vi "Main.vi"(10 "Productos Subpanel":refnum<vi>, 11 "Module Admin":refnum<class "Delacor_lib_QMH_Module Admin.lvclass">) -> ()   [LabVIEW 2020, in "Producto.lvlib"]
doc: "This template is based off of the Queued Message Handler design pattern and the Queued Message Handler project template that ships with LabVIEW.\n\nThe main difference is that the queue is private to this module and communication between modules is performed via Broadcast and Request events.\n\nRequest events are wrapped in public API methods and are handled in the Event Handling Loop (EHL) of this VI. Any module can register for Broadcast events sent by this module. The EHL generates messages based on user interface actions.\n\nThe Message Handling Loop (MHL) processes messages generated by the EHL, or by other messages. The messages are string values, so new messages can be added easily to the Message Cases case structure in the MHL. Each message cluster can also provide an optional value for Message Data, which is a variant that can be converted to whatever message-specific data is required.\n_____\nBased on Delacor QMH Project Template 5.0.0.82."
uses:
  Producto.lvlib
  <vilib>/Delacor/Delacor QMH/Libraries/Module Admin_class/Delacor_lib_QMH_Module Admin.lvclass
  Module Data--cluster.ctl
  Stop Argument--cluster.ctl
  <vilib>/Delacor/Delacor QMH/Libraries/Message Queue_class/Delacor_lib_QMH_Message Queue.lvclass/Delacor_lib_QMH_Message Queue.ctl
  <vilib>/Delacor/Delacor QMH/Libraries/Module Admin_class/Delacor_lib_QMH_Module Admin.lvclass/Delacor_lib_QMH_Module Admin.ctl
  Set Products Argument--cluster.ctl
  Actualizar inventario Argument--cluster.ctl
  <vilib>/Utility/miscctls.llb/LVPointTypeDef.ctl
  <vilib>/Delacor/Delacor QMH/Libraries/Message Queue_class/Delacor_lib_QMH_Enqueue Message (Single).vi
  <vilib>/Delacor/Delacor QMH/Libraries/Module Admin_class/Delacor_lib_QMH_Get External Launch.vi
  <vilib>/Utility/error.llb/Error Cluster From Error Code.vi
  <vilib>/ErrorRing/Error Ring.xnode
  <vilib>/Delacor/Delacor QMH/Libraries/Message Queue_class/Delacor_lib_QMH_Message Queue.lvclass
  SQLLITEDATABASE/DataBaseSQLlite.lvlib
  Monedas/Monedas.lvlib
panel:
  in  "COMPRAR BUTONN":bool
  in  "Multicolumn Listbox":i32(listbox)
  out "error out":errorcluster
  out "Status":string
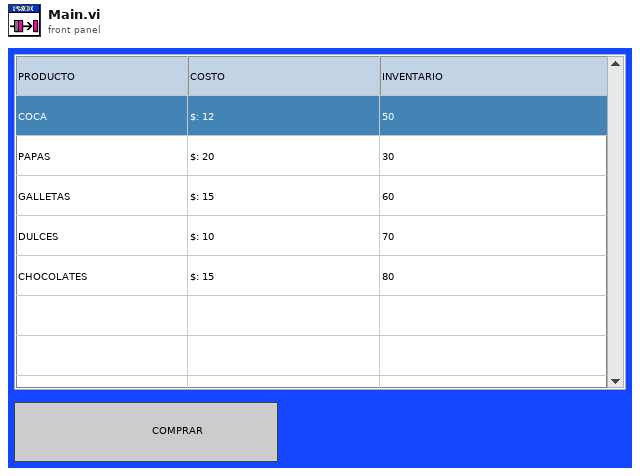
[diagram p1: front panel]
types:
  T1 = typedef "Monedas.lvlib/Broadcast Events--cluster.ctl" = cluster{"Module Did Init":refnum<user-event>, "Status Updated":refnum<user-event>, "Error Reported":refnum<user-event>, "Module Did Stop":refnum<user-event>, "Update Module Execution Status":refnum<user-event>}
  T2 = typedef "Producto.lvlib/Request Events--cluster.ctl" = cluster{"Stop Module":refnum<user-event>, "Show Panel":refnum<user-event>, "Hide Panel":refnum<user-event>, "Get Module Execution Status":refnum<user-event>, "Show Diagram":refnum<user-event>, "Set Products":refnum<user-event>, "Actualizar inventario":refnum<user-event>}
  T3 = typedef "Producto.lvlib/Module Data--cluster.ctl" = cluster{"Status":string, "PRODUCTOS EN Array":cluster{"PRODUCTO":string, "COSTO":dbl, "INVENTARIO":dbl}[], "MCListbox Refnum":refnum<vi>, "items":string[][]}
  T4 = enum32{"invalid lock state", "Not Locked", "Locked (No Password)", "Password-protected"}
  T5 = typedef "Producto.lvlib/Stop Argument--cluster.ctl" = cluster{"Origin":string, "Exit via Stop Module Req?":bool, "Wait for Module to stop?":bool}
  T6 = typedef "Producto.lvlib/Set Products Argument--cluster.ctl" = cluster{"Array":string[][]}
  T7 = typedef "Producto.lvlib/Actualizar inventario Argument--cluster.ctl" = cluster{"Boolean":bool, "Multicolumn Listbox":i32}
  T8 = typedef "LVPointTypeDef.ctl" = cluster{"Horizontal":i16, "Vertical":i16}
  T9 = enum32{"Invalid", "Standard", "Closed", "Hidden", "Minimized", "Maximized"}
  T10 = typedef "ProductInvenmtarytyppedef.ctl" = cluster{"PRODUCTO":string, "COSTO":dbl, "INVENTARIO":dbl}
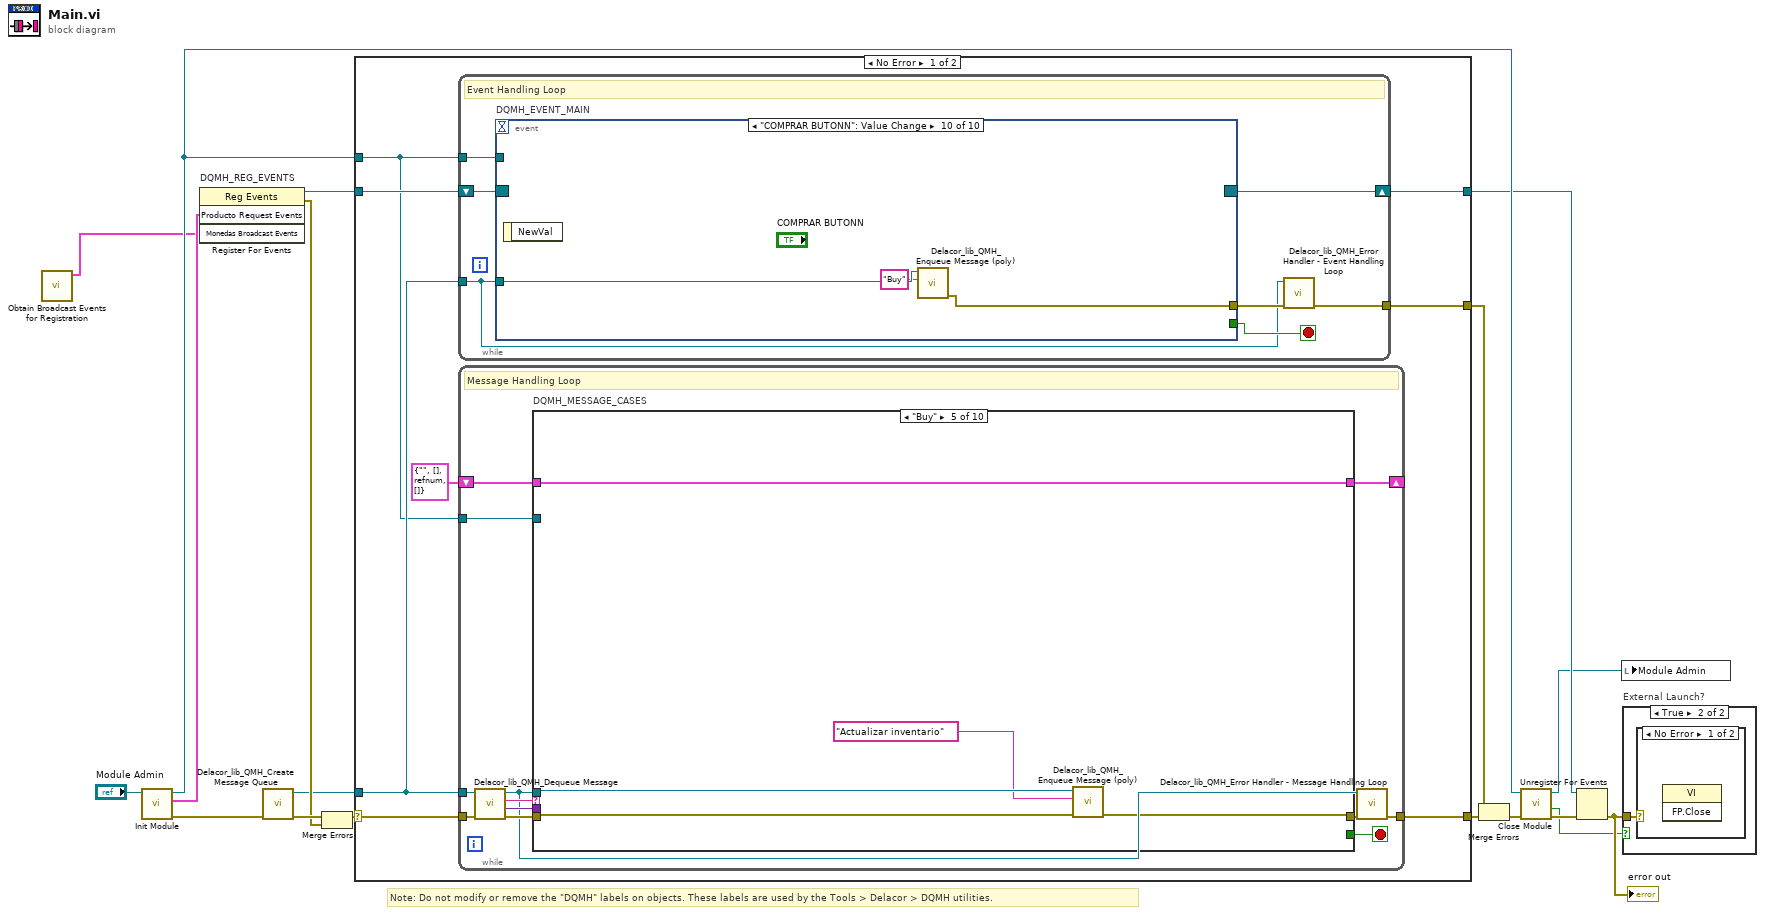
[diagram p0: block diagram]
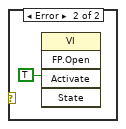
[diagram p3: hidden frame]
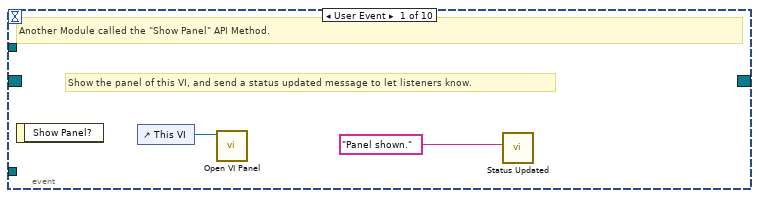
[diagram p4: hidden frame]
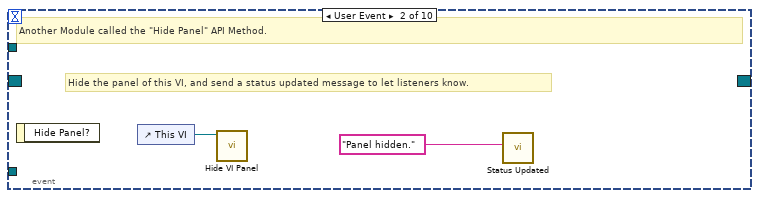
[diagram p5: hidden frame]
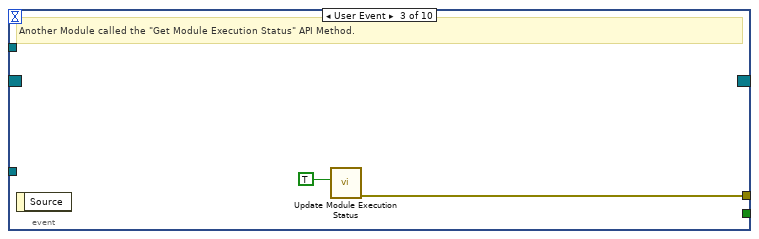
[diagram p6: hidden frame]
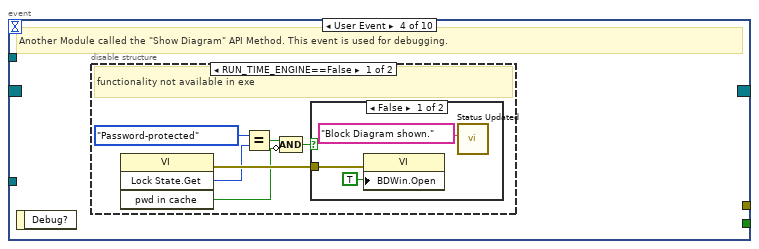
[diagram p7: hidden frame]
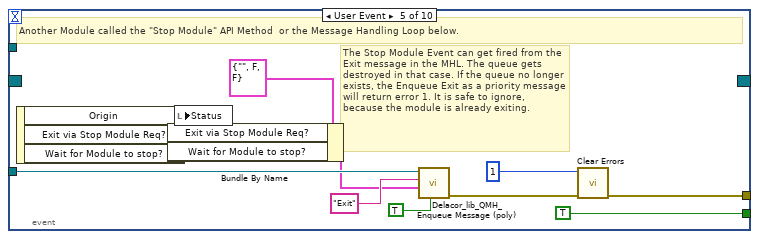
[diagram p10: hidden frame]
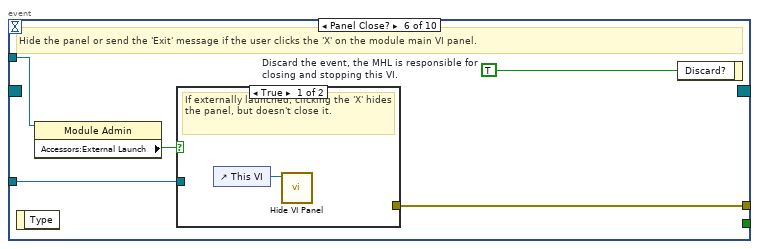
[diagram p11: hidden frame]
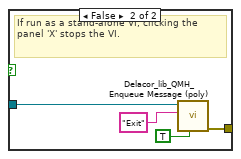
[diagram p12: hidden frame]
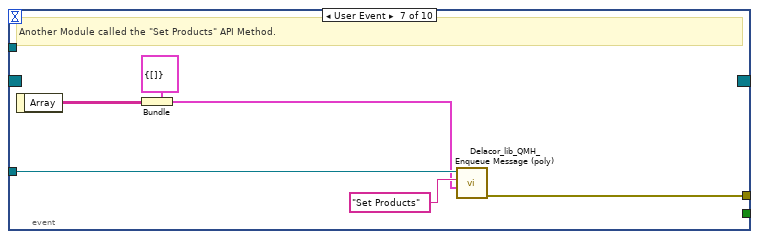
[diagram p13: hidden frame]
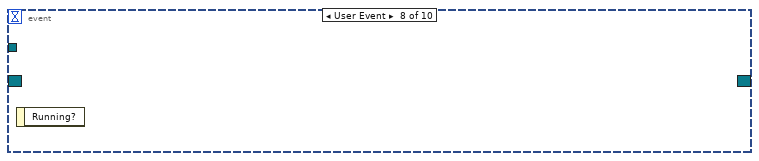
[diagram p14: hidden frame]
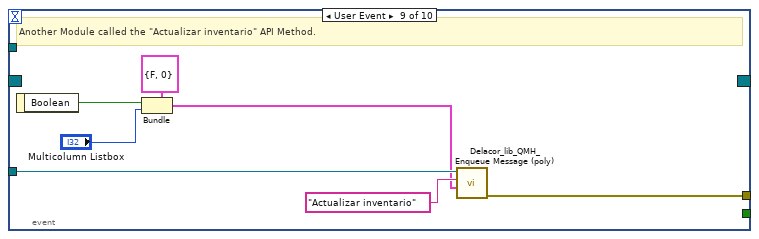
[diagram p15: hidden frame]
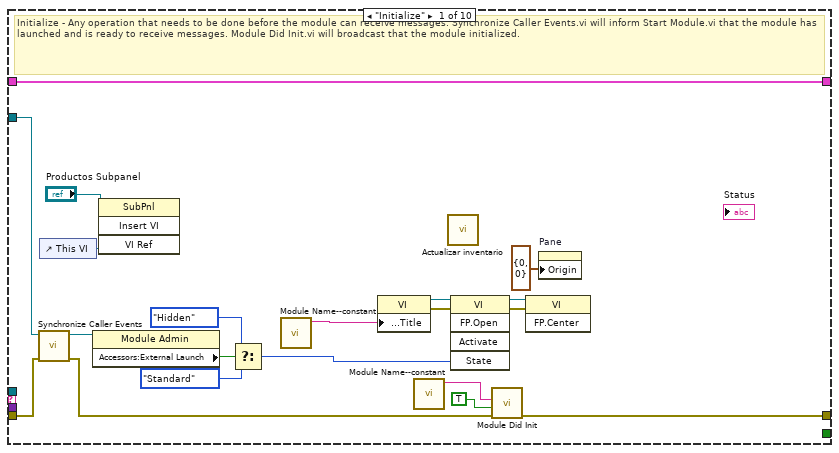
[diagram p16: hidden frame]
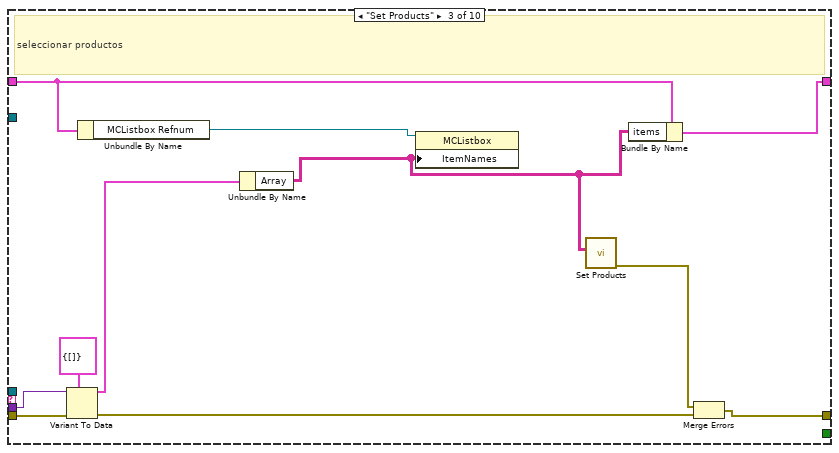
[diagram p18: hidden frame]
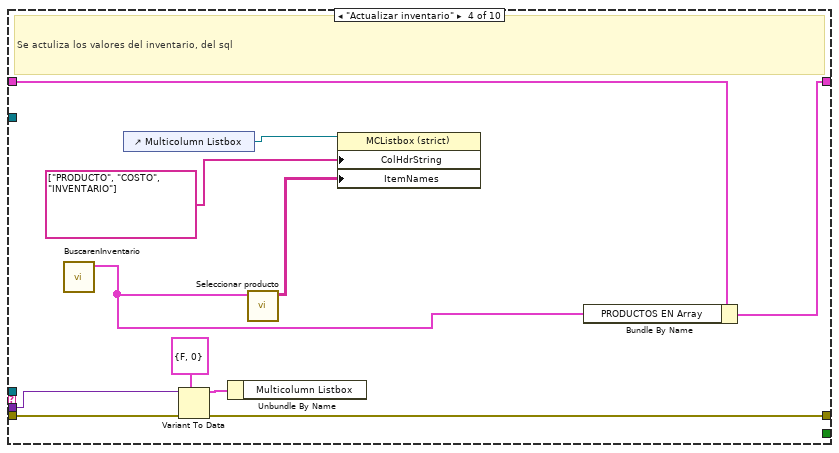
[diagram p19: hidden frame]
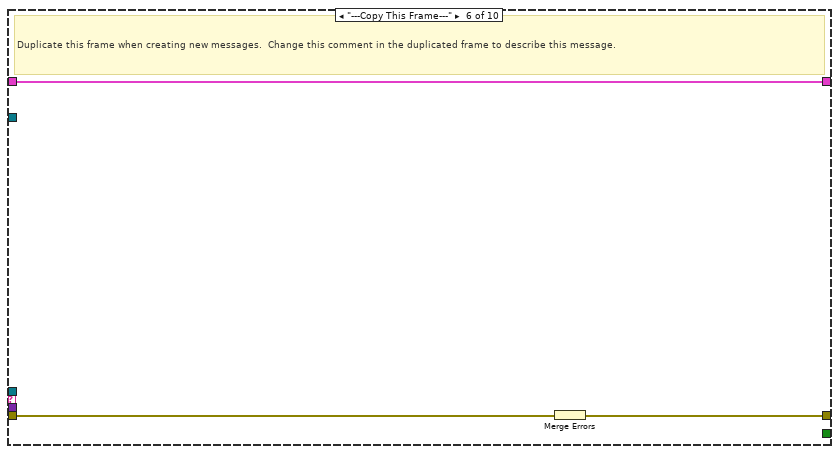
[diagram p20: hidden frame]
diagram:
  # "Note: Do not modify or remove the \"DQMH\" labels on objects. These labels are used by the Tools > Delacor > DQMH utilities."
  n1 = call "Obtain Broadcast Events for Registration.vi"() -> ("Monedas Broadcast Events"=w1:T1)  [unwired: 9 in, 2 out]
  n2 = call "Init Module.vi"("Singleton Module Admin in"="Module Admin") -> ("error out"=w17:errorcluster, "Producto Request Events"=w6:T2, "Singleton Module Admin out"=w9:refnum<class "Delacor_lib_QMH_Module Admin.lvclass">)  [unwired: 8 in]
  n3 = register-events "DQMH_REG_EVENTS"(w6, w1) -> (reference out=w7:refnum<event-registration>, error out=w10:errorcluster)  [unwired: 2 in]
  n4 = call <vilib>:"Delacor_lib_QMH_Create Message Queue.vi"("error in (no error)"=w17) -> ("error out"=w12:errorcluster, "Message Queue"=w5:refnum<class "Delacor_lib_QMH_Message Queue.lvclass">)  [unwired: 9 in]
  n5 = Merge Errors(w12, w10) -> (w11:errorcluster)
  n6 = case shown="No Error" w11 {
    selector: w11 -> [w24 w201]
    tunnel: [w26 w200] -> w18
    tunnel: [w23 w206] -> w8
    tunnel: w7 -> [w21 w206]
    tunnel: w5 -> [w20 w199]
    tunnel: [w25 _] -> w15
    tunnel: w9 -> [w19 w202]
    frame No Error {
      n7 = while {
        tunnel: w20 -> [w27]
        shift-right: [w30] -> w23
        shift-left: w21 -> [w31]
        tunnel: [w32] -> w25
        tunnel: w19 -> [w28]
        stop <- w29 stop-if-true
        # "Event Handling Loop"
        n8 = event "DQMH_EVENT_MAIN" shown="[9] \"COMPRAR BUTONN\": Value Change" {
          selector: w31 -> [_ _ _ _ _ _ _ _ _ _]
          dyn-events: [_ _ _ _ _ _ _ _ _ _] -> w30
          timeout: _ -> [_ _ _ _ _ _ _ _ _ _]
          tunnel: [_ _ _ _ TRUE ("Discard?") _ _ _ _ _] -> w29
          tunnel: w27 -> [_ _ _ _ w56 w63 w76 _ w83 w86]
          tunnel: [_ _ w39 _ w59 w65 w71 _ w78 w85] -> w33
          tunnel: w28 -> [_ _ _ _ _ w62 _ _ _ _]
          event User Event {
            # "Show the panel of this VI, and send a status updated message to let listeners know."
            # "Another Module called the \"Show Panel\" API Method."
            n9 = event-data() -> ()  [unwired: 1 in, 1 out]
            n10 = control-ref of="This VI"() -> (w35:refnum<vi>)
            n11 = call "Open VI Panel.vi"("VI"=w35) -> ()  [unwired: 10 in, 1 out]
            n12 = call "Status Updated.vi"("Status"="Panel shown." ("format string")) -> ()  [unwired: 10 in, 1 out]
          }
          event User Event {
            # "Hide the panel of this VI, and send a status updated message to let listeners know."
            # "Another Module called the \"Hide Panel\" API Method."
            n13 = event-data() -> ()  [unwired: 1 in, 1 out]
            n14 = control-ref of="This VI"() -> (w37:refnum<vi>)
            n15 = call "Hide VI Panel.vi"("VI"=w37) -> ()  [unwired: 10 in, 1 out]
            n16 = call "Status Updated.vi"("Status"="Panel hidden." ("format string")) -> ()  [unwired: 10 in, 1 out]
          }
          event User Event {
            # "Another Module called the \"Get Module Execution Status\" API Method."
            n17 = event-data() -> ()  [unwired: 1 in, 1 out]
            n18 = call "Update Module Execution Status.vi"("Running?"=TRUE) -> ("error out"=w39:errorcluster)  [unwired: 10 in]
          }
          event User Event {
            # "Another Module called the \"Show Diagram\" API Method. This event is used for debugging."
            n19 = event-data() -> ()  [unwired: 1 in, 1 out]
            n20 = disable-structure shown="RUN_TIME_ENGINE==False" {
              frame condition #0 (active) {
                # "functionality not available in exe"
                n21 = invoke class="VI" method="Lock State.Get"() -> (error out=w45:errorcluster, "Get Lock State"=w44:T4, "pwd in cache"=w41:bool)  [unwired: 4 in, 1 out]
                n22 = Equal?(x=T4."Password-protected", y=w44) -> (x = y?=w42:bool)
                n23 = Compound Arithmetic op=AND(w42, invert w41) -> (w40:bool)
                n24 = case shown="False" w40 {
                  tunnel: w45 -> [w48 _]
                  frame False {
                    n25 = property class="VI"(error in=w48, "BDWin.Open"=TRUE ("Block Diagram Window:Open")) -> ()  [unwired: 1 in, 2 out]
                    n26 = call "Status Updated.vi"("Status"="Block Diagram shown." ("format string")) -> ()  [unwired: 10 in, 1 out]
                  }
                  frame True {
                    # "Password-protected VI, and the password is not in the cache. Do not show the diagram."
                  }
                }
              }
              frame condition #1 {
              }
            }
          }
          event User Event {
            # "The Stop Module Event can get fired from the Exit message in the MHL. The queue gets destroyed in that case. If the queue no longer exists, the Enqueue Exit as a priority message will return error 1. It is safe to ignore, because the module is already exiting."
            # "Another Module called the \"Stop Module\" API Method  or the Message Handling Loop below."
            n27 = event-data() -> ("Origin"=w55:string, "Exit via Stop Module Req?"=w51:bool, "Wait for Module to stop?"=w50:bool)  [unwired: 1 in]
            n28 = Bundle By Name(cluster=T5 {"Origin"="", "Exit via Stop Module Req?"=FALSE, "Wait for Module to stop?"=FALSE} ("Stop Argument"), "Exit via Stop Module Req?"=w51, "Wait for Module to stop?"=w50) -> (w49:T5)
            n29 = local write "Status"(w55) -> ()
            n30 = call-poly <vilib>:"Delacor_lib_QMH_Enqueue Message (poly).vi"("Priority Message? (F)"=TRUE, "Message Data"=w49, "Message"="Exit", "Message Queue in"=w56) -> ("error out"=w60:errorcluster)  [unwired: 6 in, 1 out]
            n31 = call <vilib>:"Clear Errors.vi"("error in (no error)"=w60, "specific error code to clear (0: all)"=1) -> ("error out"=w59:errorcluster)  [unwired: 4 in, 1 out]
          }
          event Panel Close? {
            w64 = TRUE  # Discard the event, the MHL is responsible for closing and stopping this VI.
            # "Hide the panel or send the 'Exit' message if the user clicks the 'X' on the module main VI panel."
            n32 = event-data() -> ()  [unwired: 1 in, 1 out]
            n33 = property class="Module Admin"(reference=w62) -> ("Accessors:External Launch"=w61:bool)  [unwired: 1 in, 2 out]
            n34 = case shown="True" w61 {
              tunnel: w63 -> [_ w69]
              tunnel: [_ w70] -> w65
              frame True {
                # "If externally launched, clicking the 'X' hides the panel, but doesn't close it."
                n35 = control-ref of="This VI"() -> (w66:refnum<vi>)
                n36 = call "Hide VI Panel.vi"("VI"=w66) -> ()  [unwired: 10 in, 1 out]
              }
              frame False {
                # "If run as a stand-alone VI, clicking the panel 'X' stops the VI."
                n37 = call-poly <vilib>:"Delacor_lib_QMH_Enqueue Message (poly).vi"("Priority Message? (F)"=TRUE, "Message"="Exit", "Message Queue in"=w69) -> ("error out"=w70:errorcluster)  [unwired: 7 in, 1 out]
              }
            }
            n38 = event-data("Discard?"=w64) -> ()  [unwired: 1 in, 1 out]
          }
          event User Event {
            # "Another Module called the \"Set Products\" API Method."
            n39 = event-data() -> ("Array"=w72:string[][])  [unwired: 1 in]
            n40 = Bundle(cluster=T6 {"Array"=[]} ("Set Products Argument"), "Array"=w72) -> (w73:T6)
            n41 = call-poly <vilib>:"Delacor_lib_QMH_Enqueue Message (poly).vi"("Message Data"=w73, "Message"="Set Products", "Message Queue in"=w76) -> ("error out"=w71:errorcluster)  [unwired: 7 in, 1 out]
          }
          event User Event {
            n42 = event-data() -> ()  [unwired: 1 in, 1 out]
          }
          event User Event {
            # "Another Module called the \"Actualizar inventario\" API Method."
            n43 = event-data() -> ("Boolean"=w79:bool)  [unwired: 1 in]
            n44 = Bundle(cluster=T7 {"Boolean"=FALSE, "Multicolumn Listbox"=0} ("Actualizar inventario Argument"), "Boolean"=w79, "Multicolumn Listbox"="Multicolumn Listbox") -> (w80:T7)
            n45 = call-poly <vilib>:"Delacor_lib_QMH_Enqueue Message (poly).vi"("Message Data"=w80, "Message"="Actualizar inventario", "Message Queue in"=w83) -> ("error out"=w78:errorcluster)  [unwired: 7 in, 1 out]
          }
          event "COMPRAR BUTONN": Value Change {
            n46 = event-data() -> ()  [unwired: 1 in, 1 out]
            n47 = call-poly <vilib>:"Delacor_lib_QMH_Enqueue Message (poly).vi"("Message"="Buy", "Message Queue in"=w86) -> ("error out"=w85:errorcluster)  [unwired: 8 in, 1 out]
          }
        }
        n48 = call-dynamic "Delacor_lib_QMH_Error Handler - Event Handling Loop.vi"("error in (no error)"=w33, "Message Queue in"=w27) -> ("dup error in"=w32:errorcluster)  [unwired: 8 in, 1 out]
      }
      n49 = while {
        tunnel: w20 -> [w89]
        shift-right: [w93] -> _
        shift-left: T3 {"Status"="", "PRODUCTOS EN Array"=[], "MCListbox Refnum"=refnum, "items"=[]} ("Data Cluster") -> [w94]
        tunnel: w24 -> [w97]
        tunnel: [w95] -> w26
        tunnel: w19 -> [w87]
        stop <- w92 stop-if-true
        # "Message Handling Loop"
        n50 = call-dynamic "Delacor_lib_QMH_Dequeue Message.vi"("error in (no error)"=w97, "Message Queue in"=w89) -> ("error out"=w96:errorcluster, "Message Data"=w90:variant, "Message"=w91:string, "Message Queue out"=w88:refnum<class "Delacor_lib_QMH_Message Queue.lvclass">)  [unwired: 6 in]
        n51 = case "DQMH_MESSAGE_CASES" shown="\"Buy\"" w91 {
          selector: w91 -> [_ _ _ _ _ _ _ _ _ w186]
          tunnel: w88 -> [_ _ _ _ w144 _ _ w156 w178 _]
          tunnel: w96 -> [w116 w120 w131 w142 w145 w150 w152 w163 w184 w188]
          tunnel: [w114 w120 w123 w141 w146 w149 w152 w159 w181 w189] -> w98
          tunnel: w94 -> [w105 w119 w126 w132 w147 w148 w151 w158 w177 w187]
          tunnel: [w105 w119 w125 w134 w147 w148 w151 w158 w177 w187] -> w93
          tunnel: [_ _ _ _ _ _ _ _ w176 _] -> w92
          tunnel: w90 -> [_ _ w130 w140 _ _ _ w157 w175 _]
          tunnel: w87 -> [w106 _ _ _ _ _ _ w155 w170 _]
          frame "Initialize" {
            # "Initialize - Any operation that needs to be done before the module can receive messages. Synchronize Caller Events.vi will inform Start Module.vi that the module has launched and is ready to receive messages. Module Did Init.vi will broadcast that the module initialized."
            n52 = call "Synchronize Caller Events.vi"("error in (no error)"=w116, "Singleton Module Admin in"=w106) -> ("error out"=w115:errorcluster, "Singleton Module Admin out"=w102:refnum<class "Delacor_lib_QMH_Module Admin.lvclass">)  [unwired: 8 in]
            n53 = control-ref of="This VI"() -> (w99:refnum<vi>)
            n54 = property class="Module Admin"(reference=w102) -> ("Accessors:External Launch"=w110:bool)  [unwired: 1 in, 2 out]
            n55 = invoke class="SubPnl" method="Insert VI"(reference="Productos Subpanel", "VI Ref"=w99) -> ()  [unwired: 2 in, 4 out]
            n56 = Select(t=T9."Hidden" ("State"), s=w110, f=T9."Standard" ("State")) -> (s? t:f=w107:T9)
            n57 = call "Module Name--constant.vi"() -> ("Module Name"=w113:string)  [unwired: 11 in]
            n58 = property class="VI"("Front Panel.Title"=w113) -> (reference out=w112:refnum<vi>, error out=w118:errorcluster)  [unwired: 2 in]
            n59 = call "Module Name--constant.vi"() -> ("Module Name"=w103:string)  [unwired: 11 in]
            n60 = call "Actualizar inventario.vi"() -> ()  [unwired: 11 in, 1 out]
            n61 = invoke class="VI" method="FP.Open"(reference=w112, error in=w118, "State"=w107) -> (reference out=w111:refnum<vi>, error out=w117:errorcluster)  [unwired: 2 in, 3 out]
            n62 = call "Module Did Init.vi"("error in (no error)"=w115, "Initialized?"=TRUE, "Origin"=w103) -> ("error out"=w114:errorcluster)  [unwired: 8 in]
            n63 = invoke class="VI" method="FP.Center"(reference=w111, error in=w117) -> ()  [unwired: 1 in, 3 out]
            n64 = property on="Pane" class="Pane"("Origin"=T8 {"Horizontal"=0, "Vertical"=0}) -> ()  [unwired: 2 in, 2 out]
          }
          frame "--- Module Specific ---" {
            # "Separator -- The following cases handle messages specific to this Module."
          }
          frame "Set Products" {
            # "seleccionar productos"
            n65 = Variant To Data(error in=w131, type=T6 {"Array"=[]} ("Set Products Argument"), Variant=w130) -> (data=w128:T6, error out=w122:errorcluster)
            n66 = Unbundle By Name(w126) -> ("MCListbox Refnum"=w127:refnum<vi>)
            n67 = Unbundle By Name(w128) -> ("Array"=w124:string[][])
            n68 = property class="MCListbox"(reference=w127, "ItemNames"=w124) -> ()  [unwired: 1 in, 2 out]
            n69 = call "Set Products.vi"("Array"=w124) -> ("error out"=w121:errorcluster)  [unwired: 10 in]
            n70 = Bundle By Name(cluster=w126, "items"=w124) -> (w125:T3)
            n71 = Merge Errors(w121, w122) -> (w123:errorcluster)
          }
          frame "Actualizar inventario" {
            # "Se actuliza los valores del inventario, del sql"
            n72 = call "BuscarenInventario.vi"() -> ("Array"=w133:T10[])  [unwired: 10 in, 1 out]
            n73 = control-ref of="Multicolumn Listbox"() -> (w137:refnum<vi>)
            n74 = Variant To Data(error in=w142, type=T7 {"Boolean"=FALSE, "Multicolumn Listbox"=0} ("Actualizar inventario Argument"), Variant=w140) -> (data=w138:T7, error out=w141:errorcluster)
            n75 = Unbundle By Name(w138) -> ()  [unwired: 1 out]
            n76 = call "Seleccionar producto.vi"("PRODUCTOS EN Array"=w133) -> ("Array"=w135:string[][])  [unwired: 10 in]
            n77 = property class="MCListbox (strict)"(reference=w137, "ColHdrString"=string[] ["PRODUCTO", "COSTO", "INVENTARIO"], "ItemNames"=w135) -> ()  [unwired: 1 in, 2 out]
            n78 = Bundle By Name(cluster=w132, "PRODUCTOS EN Array"=w133) -> (w134:T3)
          }
          frame "Buy" {
            n79 = call-poly <vilib>:"Delacor_lib_QMH_Enqueue Message (poly).vi"("error in (no error)"=w145, "Message"="Actualizar inventario", "Message Queue in"=w144) -> ("error out"=w146:errorcluster)  [unwired: 7 in, 1 out]
          }
          frame "---Copy This Frame---" {
            # "Duplicate this frame when creating new messages.  Change this comment in the duplicated frame to describe this message."
            n80 = Merge Errors(w150) -> (w149:errorcluster)
          }
          frame "--- Exit and Error Handling---" {
            # "Separator - The following cases handle errors and exit messages."
          }
          frame "Error" {
            # "#CodeRecommended - If you ever change the name of this \"Error\" message, you'll need to update the name in the Check Loop Error.vi as well."
            # "#CodeRecommended - If the module is running in standalone mode (External Launch = FALSE), this code will pop up an error dialog and call the 'Exit' message if an error occurs. Add more fine-grained error handling here."
            # "Error - Check the error message data and respond accordingly. This message is sent by the \"Error Handler\" VIs at the end of each loop in this application."
            n81 = property class="Module Admin"(reference=w155) -> ("Accessors:External Launch"=w154:bool)  [unwired: 1 in, 2 out]
            n82 = Variant To Data(error in=w163, type=errorcluster {"status"=FALSE, "code"=0, "source"=""} ("error constant"), Variant=w157) -> (data=w164:errorcluster, error out=w161:errorcluster)
            n83 = call "Module Name--constant.vi"() -> ("Module Name"=w153:string)  [unwired: 11 in]
            n84 = call "Error Reported.vi"("Additional Information"=w153, "Error"=w164) -> ()  [unwired: 9 in, 1 out]
            n85 = case shown="False" w154 {
              tunnel: [w169 _] -> w160
              tunnel: w156 -> [w167 _]
              tunnel: w164 -> [w168 _]
              frame False {
                # "If the module is running standalone, then pop up an error dialog and call the \"Exit\" message."
                n86 = call <vilib>:"Simple Error Handler.vi"("error in (no error)"=w168) -> ()  [unwired: 4 in, 5 out]
                n87 = call-poly <vilib>:"Delacor_lib_QMH_Enqueue Message (poly).vi"("Priority Message? (F)"=TRUE, "Message"="Exit", "Message Queue in"=w167) -> ("error out"=w169:errorcluster)  [unwired: 7 in, 1 out]
              }
              frame True {
                # "If the module was launched externally, calling the Error Reported broadcast VI is the only action performed by the \"Error\" message. The module's caller can then process the error appropriately."
              }
            }
            n88 = Merge Errors(w161, w160) -> (w159:errorcluster)
            n89 = local write "error out"(w159) -> ()
          }
          frame "Exit" {
            w174 = 91  # 91: not all Exit messages will have an argument
            w176 = TRUE  # Stop the VI
            # "Release the message queue reference"
            # "#CodeNeeded - Add any required cleanup code here"
            # "Exit - Exit the application."
            n90 = Variant To Data(error in=w184, type=T5 {"Origin"="", "Exit via Stop Module Req?"=FALSE, "Wait for Module to stop?"=FALSE} ("Stop Argument"), Variant=w175) -> (data=w172:T5, error out=w180:errorcluster)
            n91 = call <vilib>:"Clear Errors.vi"("error in (no error)"=w180, "specific error code to clear (0: all)"=w174) -> ("error out"=w183:errorcluster)  [unwired: 4 in, 1 out]
            n92 = control-ref of="This VI"() -> (w171:refnum<vi>)
            n93 = call-dynamic "Delacor_lib_QMH_Release Message Queue.vi"("error in (no error)"=w183, "Message Queue"=w178) -> ("error out"=w182:errorcluster)  [unwired: 9 in]
            n94 = call "Handle Exit.vi"("Stop Argument"=w172, "Admin in"=w170, "VI reference"=w171) -> ("error out"=w179:errorcluster)  [unwired: 7 in, 1 out]
            n95 = Merge Errors(w182, w179) -> (w181:errorcluster)
          }
          frame Default {
            # "'Default' case only runs if there is a message that isn't defined in any of the other cases.  Output a programming error."
            n96 = call "Module Name--constant.vi"() -> ("Module Name"=w185:string)  [unwired: 11 in]
            n97 = xnode "Error Ring"("parameter 0"=w186, "parameter 1"=w185) -> ("error out"=w190:errorcluster)
            n98 = Merge Errors(w188, w190) -> (w189:errorcluster)
          }
        }
        n99 = call-dynamic "Delacor_lib_QMH_Error Handler - Message Handling Loop.vi"("error in (no error)"=w98, "Message Queue in"=w88) -> ("dup error in"=w95:errorcluster)  [unwired: 8 in, 1 out]
      }
    }
    frame Error {
      # "Synchronize Caller Events.vi will inform Start Module.vi that the module has launched and will let the code calling Start Module.vi register for broadcasts and would permit the caller receive the broadcast that an error occurred at launch time."
      n100 = call-dynamic "Delacor_lib_QMH_Release Message Queue.vi"("error in (no error)"=w201, "Message Queue"=w199) -> ("error out"=w200:errorcluster)  [unwired: 9 in]
      n101 = call "Synchronize Caller Events.vi"("Singleton Module Admin in"=w202) -> ("error out"=w207:errorcluster)  [unwired: 9 in, 1 out]
      n102 = call "Module Name--constant.vi"() -> ("Module Name"=w205:string)  [unwired: 11 in]
      n103 = Format Into String(format string="An error occurred during initialization. %s is no longer running.", w205) -> (resulting string=w203:string)  [unwired: 2 in, 1 out]
      n104 = Merge Errors(w200, w207) -> (w208:errorcluster)
      n105 = call "Error Reported.vi"("Additional Information"=w203, "Error"=w208) -> ()  [unwired: 9 in, 1 out]
    }
  }
  n106 = Merge Errors(w15, w18) -> (w14:errorcluster)
  n107 = call "Close Module.vi"("error in (no error)"=w14, "Module Admin in"=w9) -> ("error out"=w16:errorcluster, "External Launch"=w2:bool, "Module Admin out"=w3:refnum<class "Delacor_lib_QMH_Module Admin.lvclass">)  [unwired: 7 in]
  n108 = Unregister For Events(event registration refnum=w8, error in=w16) -> (error out=w13:errorcluster)
  "error out" <- w13
  n109 = local write "Module Admin"(w3) -> ()
  n110 = case "External Launch?" shown="True" w2 {
    tunnel: w13 -> [_ w209]
    frame False {
    }
    frame True {
      n111 = case shown="No Error" w209 {
        frame No Error {
          n112 = invoke class="VI" method="FP.Close"() -> ()  [unwired: 3 in, 3 out]
        }
        frame Error {
          n113 = invoke class="VI" method="FP.Open"("Activate"=TRUE ("Activate?")) -> ()  [unwired: 4 in, 5 out]
        }
      }
    }
  }
